vi "UpdateVI.vi"(8 "error in (no error)":errorcluster, 10 "Controls":path, 11 "VIToUpdate":path) -> (0 "error out":errorcluster, 3 "reference out":refnum<vi>)   [LabVIEW 2016]
uses:
  <vilib>/Utility/traverseref.llb/TRef TravTarget.ctl
  <vilib>/Utility/traverseref.llb/VI Scripting - Traverse.lvlib
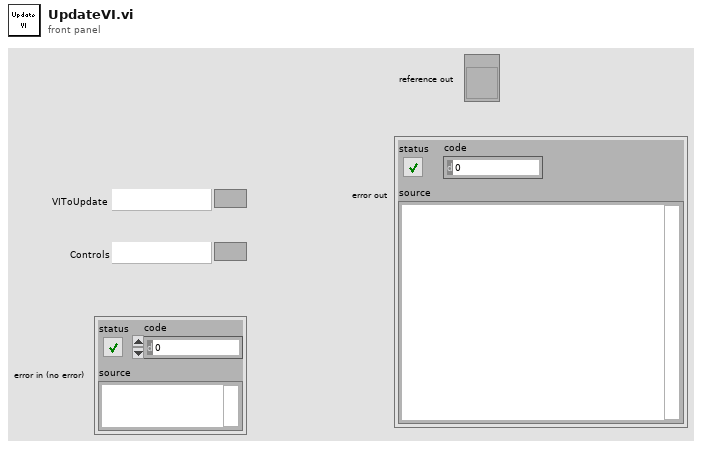
[diagram p1: front panel]
types:
  T1 = typedef "TRef TravTarget.ctl" = enum16{"FP", "BD", "Other"}
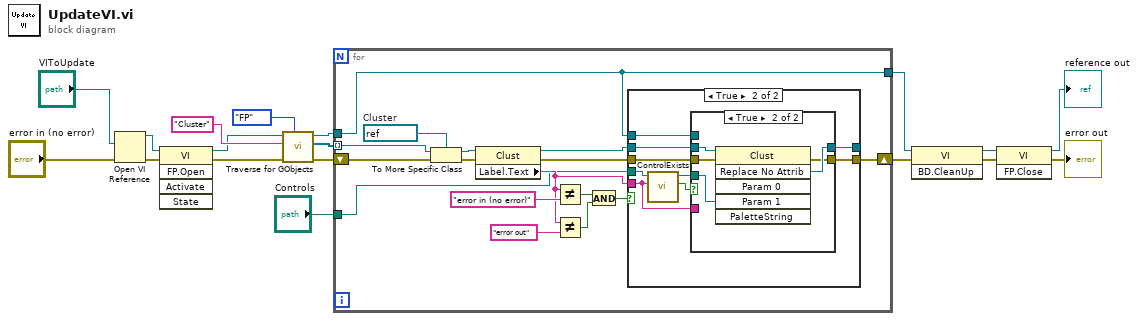
[diagram p0: block diagram]
diagram:
  n1 = Open VI Reference(vi path="VIToUpdate", error in (no error)="error in (no error)") -> (vi reference=w12:refnum<vi>, error out=w8:errorcluster)  [unwired: 4 in]
  n2 = invoke class="VI" method="FP.Open"(reference=w12, error in=w8) -> (reference out=w9:refnum<vi>, error out=w7:errorcluster)  [unwired: 3 in, 3 out]
  n3 = call <vilib>:"Traverse for GObjects.vi"("Traverse Target"=TRef_TravTarget."FP", "error in (no error)"=w7, "Class Name"="Cluster", "VI Refnum"=w9) -> ("error out"=w14:errorcluster, "References"=w16:refnum<vi>[], "dup VI Refnum"=w15:refnum<vi>)  [unwired: 4 in, 1 out]
  n4 = for {
    tunnel: w16 -> [w32] mode=indexing
    tunnel: w15 -> [w20]
    shift-right: [w19] -> w2
    shift-left: w14 -> [w33]
    tunnel: "Controls" -> [w21]
    tunnel: [w20] -> w3
    w34 = refnum<vi> refnum  # Cluster
    n5 = To More Specific Class(target class=w34, reference=w32, error in=w33) -> (specific class reference=w31:refnum<vi>, error out=w30:errorcluster)
    n6 = property class="Clust"(reference=w31, error in=w30) -> (reference out=w22:refnum<vi>, error out=w24:errorcluster, "Label.Text"=w23:string)
    n7 = Not Equal?(x=w23, y="error in (no error)") -> (x != y?=w28:bool)
    n8 = Not Equal?(x=w23, y="error out") -> (x != y?=w29:bool)
    n9 = And(x=w28, y=w29) -> (x .and. y?=w25:bool)
    n10 = case shown="True" w25 {
      tunnel: w24 -> [w35 w45]
      tunnel: w23 -> [_ w40]
      tunnel: w22 -> [w36 w44]
      tunnel: [w35 w43] -> w19
      tunnel: [w36 w42] -> _
      tunnel: w21 -> [_ w41]
      tunnel: w20 -> [_ w37]
      frame False {
      }
      frame True {
        n11 = call "ControlExists.vi"("ControlName"=w40, "ControlsPath"=w41) -> ("Boolean"=w39:bool, "ControlPath"=w38:path)  [unwired: 8 in]
        n12 = case shown="True" w39 {
          tunnel: w45 -> [w47 w50]
          tunnel: w44 -> [w46 w51]
          tunnel: [w47 w48] -> w43
          tunnel: [w46 w49] -> w42
          tunnel: w40 -> [_ _]
          tunnel: w38 -> [_ w52]
          tunnel: w37 -> [_ _]
          frame False {
          }
          frame True {
            n13 = invoke class="Clust" method="Replace No Attrib"(reference=w51, error in=w50, "Param 1"=w52) -> (error out=w48:errorcluster, "RepNoAttrib"=w49:refnum<vi>)  [unwired: 3 in, 4 out]
          }
        }
      }
    }
  }
  n14 = invoke class="VI" method="BD.CleanUp"(reference=w3, error in=w2) -> (reference out=w11:refnum<vi>, error out=w10:errorcluster)  [unwired: 1 in, 1 out]
  n15 = invoke class="VI" method="FP.Close"(reference=w11, error in=w10) -> (reference out=→"reference out":refnum<vi>, error out=→"error out":errorcluster)  [unwired: 1 in, 1 out]
